vi "PH_HamamatsuCamera.State Configure.vi"(0 "VI in":refnum<vi>, 1 "Parameter changed":bool, 2 "ROI changed":bool, 3 "Trigger Sets changed":bool, 5 "error in (no error)":errorcluster) -> (14 "VI out":refnum<vi>, 15 "Cam Handle out":i32, 18 "Cam Error":errorcluster, 19 "error out":errorcluster)   [LabVIEW 2014, in "PH_HamamatsuCamera.lvlib"]
uses:
  PH_HamamatsuCamera.lvlib
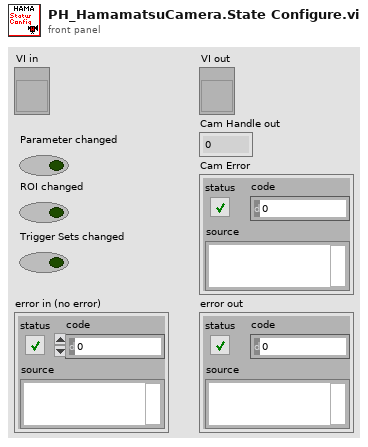
[diagram p1: front panel]
types:
  T1 = typedef "PH_HamamatsuCamera.lvlib/PH_HamamatsuCamera.i attribute.ctl" = cluster{"Gui Refs":cluster{"Camera Details":refnum<vi>, "ROI":refnum<vi>, "Set ROI to Maximum":refnum<vi>, "Trigger Parameters":refnum<vi>, "Brightness":refnum<vi>, "Shutter":refnum<vi>, "Gain":refnum<vi>, "Trigger Timeout":refnum<vi>, "Trigger Polarity":refnum<vi>, "Trigger Mode":refnum<vi>, "Parameters":refnum<vi>, "Set Cam Parameter":refnum<vi>, "Parameter to set":refnum<vi>, "Value to set":refnum<vi>}, "Cam":cluster{"Handle":i32, "Details":cluster{"Model":string, "Camera ID":string, "Firmware":string}, "Buffer Info":cluster{"height":u32, "width":u32, "datatype":u32}}, "H Offset":cluster{"Value":i32, "Minimum":i32, "Maximum":i32, "Increment":i32}, "V Offset":cluster{"Value":i32, "Minimum":i32, "Maximum":i32, "Increment":i32}, "H Width":cluster{"Value":i32, "Minimum":i32, "Maximum":i32, "Increment":i32}, "V Width":cluster{"Value":i32, "Minimum":i32, "Maximum":i32, "Increment":i32}, "Trigger Parameters":T2, "Trigger Timeout":u32, "Parameters":T3[], "Indicees Cam Parameters":cluster{"Brightness":i32, "Shutter":i32, "Gain":i32}, "Wanted Values":cluster{"Trigger Settings":T2[], "ROI":T4[], "Parameter":cluster{"Name":string, "Value":dbl}[]}}
  T2 = typedef "PH_HamamatsuCamera.lvlib/PH_HamamatsuCamera.Trigger Parameter.ctl" = cluster{"Mode":u32, "Polarity":u32, "Times":u32, "Delay":dbl}
  T3 = typedef "PH_HamamatsuCamera.lvlib/PH_HamamatsuCamera.Parameter Set.ctl" = cluster{"Parameter":string, "Value":dbl, "Writable":bool, "Range":cluster{"min":dbl, "max":dbl, "step":dbl}, "Default":dbl, "Value Names":cluster{"Name":string, "Value":dbl}[], "Text Values":bool}
  T4 = typedef "PH_HamamatsuCamera.lvlib/PH_HamamatsuCamera.ROI.ctl" = cluster{"Horizontal Offset":i32, "Vertical Offset":i32, "Horizontal Width":i32, "Vertical Width":i32}
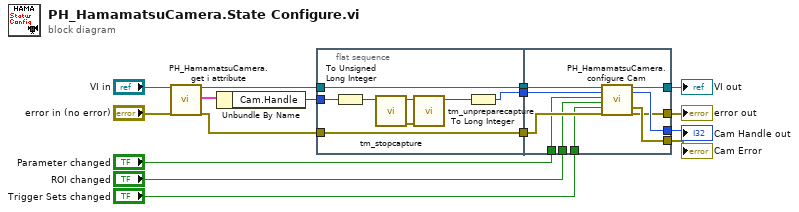
[diagram p0: block diagram]
diagram:
  n1 = call "PH_HamamatsuCamera.get i attribute.vi"("i ref in"="VI in", "error in (no error)"="error in (no error)") -> ("i ref out"=w5:refnum<vi>, "i attribute"=w7:T1, "error out"=w8:errorcluster)  [unwired: 15 in]
  n2 = Unbundle By Name(w7) -> ("Cam.Handle"=w4:i32)
  n3 = flat-sequence {
    tunnel: w4 -> [w17]
    tunnel: w8 -> [w23]
    tunnel: w5 -> [w24]
    tunnel: [w24] -> w12
    tunnel: [w23] -> w11
    tunnel: [w18] -> w10
    tunnel: [w29] -> w16
    tunnel: [w28] -> w15
    tunnel: [w34] -> w14
    tunnel: [w31] -> w13
    tunnel: w12 -> [w33]
    tunnel: w11 -> [w32]
    tunnel: w10 -> [w30]
    tunnel: "Parameter changed" -> [w27]
    tunnel: "ROI changed" -> [w26]
    tunnel: "Trigger Sets changed" -> [w25]
    frame #0 {
      n4 = To Unsigned Long Integer(number=w17) -> (unsigned 32bit integer=w22:u32)
      n5 = call <userlib>:"tm_stopcapture.vi"("Handle in"=w22) -> ("error out"=w20:errorcluster, "Handle out"=w21:u32)  [unwired: 9 in]
      n6 = call <userlib>:"tm_unpreparecapture.vi"("error in (no error)"=w20, "Handle in"=w21) -> ("Handle out"=w19:u32)  [unwired: 8 in, 1 out]
      n7 = To Long Integer(number=w19) -> (32bit integer=w18:i32)
    }
    frame #1 {
      n8 = call "PH_HamamatsuCamera.configure Cam.vi"("VI in"=w33, "Cam Handle in"=w30, "Parameter changed"=w27, "ROI changed"=w26, "Trigger Sets changed"=w25, "error in (no error)"=w32) -> ("VI out"=w29:refnum<vi>, "Cam Handle out"=w31:i32, "Cam Error out"=w34:errorcluster, "error out"=w28:errorcluster)  [unwired: 10 in]
    }
  }
  "Cam Error" <- w14
  "error out" <- w15
  "VI out" <- w16
  "Cam Handle out" <- w13
